vi "oa_TV Differentiator (1Chan).vi"(5 "reset? (True)":bool=TRUE, 8 "error in (no error)":errorcluster, 10 "deltaX":dbl=1.0 format="%.2f", 11 "Y[n]":dbl[](array[numeric]) format="%.2f") -> (0 "error out":errorcluster, 1 "Delay":dbl, 2 "X[n]":dbl[](array[numeric]) format="%.2f", 3 "dY[n]/dX[n]":dbl[](array[numeric]) format="%.2f")   [LabVIEW 2017, in "SoundVib_Torsional.lvlib"]
uses:
  <vilib>/addons/Sound and Vibration/Order Analysis/Torsional Vibration/SoundVib_Torsional.lvlib
  <vilib>/Analysis/3filter.llb/FIR Filter with I.C. (DBL).vi
  <vilib>/Analysis/NI_AALBase.lvlib
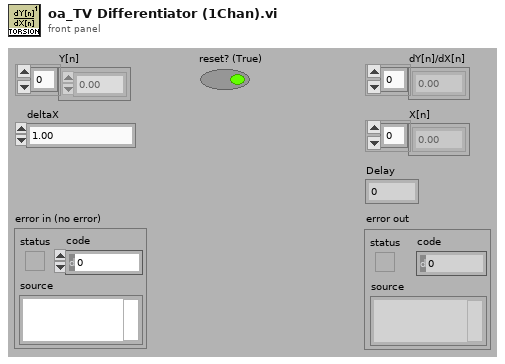
[diagram p1: front panel]
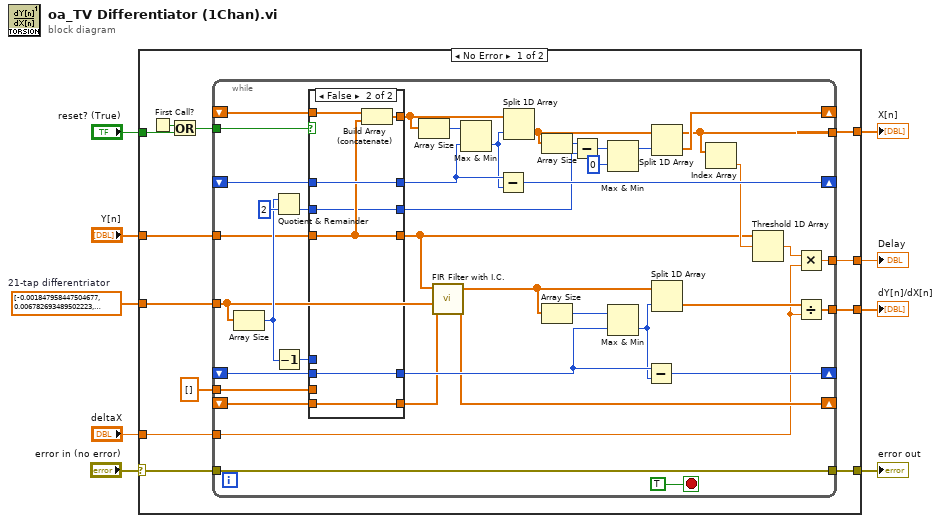
[diagram p0: block diagram]
diagram:
  w3 = dbl[] [-0.001847958447504677, 0.006782693489502223, -0.015759314785292692, 0.03157696398653407, -0.05723345514019107, 0.09716912388312568, -0.15901162473423236, 0.2593879138454093, -0.4476586474107506, 0.9725301910180191, 0.0, -0.9725301910180191, 0.4476586474107506, -0.2593879138454093, 0.15901162473423236, -0.09716912388312568, 0.05723345514019107, -0.03157696398653407, 0.015759314785292692, -0.006782693489502223, 0.001847958447504677]  # 21-tap differentriator
  n1 = case shown="No Error" "error in (no error)" {
    selector: "error in (no error)" -> [w20 w75]
    tunnel: [w17 w75] -> w9
    tunnel: [w21 _] -> w8
    tunnel: [w13 _] -> w7
    tunnel: "Y[n]" -> [w12 _]
    tunnel: w3 -> [w19 _]
    tunnel: "reset? (True)" -> [w16 _]
    tunnel: [w11 0.0] -> w2
    tunnel: "deltaX" -> [w10 _]
    frame No Error {
      n2 = First Call?() -> (First Call?: T/F=w15:bool)
      n3 = Or(x=w15, y=w16) -> (x .or. y?=w14:bool)
      n4 = while {
        tunnel: [w62] -> w21
        tunnel: w20 -> [w31]
        tunnel: w19 -> [w35]
        shift-right: [w32] -> _
        shift-left: _ -> [w60]
        shift-right: [w49] -> _
        shift-left: _ -> [w47]
        shift-right: [w55] -> _
        shift-left: _ -> [w54]
        tunnel: w14 -> [w30]
        tunnel: [w25] -> w13
        shift-right: [w40] -> _
        shift-left: _ -> [w45]
        tunnel: dbl[] [] ("t") -> [w37]
        tunnel: [w31] -> w17
        tunnel: w12 -> [w33]
        tunnel: [w23] -> w11
        tunnel: w10 -> [w22]
        stop <- TRUE stop-if-true
        n5 = Array Size(array=w35) -> (size(s)=w39:i32)
        n6 = Quotient & Remainder(x=w39, y=2) -> (floor(x/y)=w36:i32)  [unwired: 1 out]
        n7 = Decrement(x=w39) -> (x-1=w46:i32)
        n8 = case shown="False" w30 {
          tunnel: w60 -> [_ w71]
          tunnel: [w63 w69] -> w57
          tunnel: w54 -> [_ w69]
          tunnel: [w64 w73] -> w48
          tunnel: w47 -> [_ w72]
          tunnel: w46 -> [w66 _]
          tunnel: w45 -> [_ w70]
          tunnel: [w66 w70] -> w42
          tunnel: w37 -> [w65 _]
          tunnel: w36 -> [w63 w67]
          tunnel: [w65 w71] -> w34
          tunnel: w33 -> [w64 w68]
          tunnel: [w64 w68] -> w26
          tunnel: [w63 w67] -> w29
          frame True {
          }
          frame False {
            n9 = Build Array (concatenate)(w72, w68) -> (w73:dbl[])
          }
        }
        n10 = Array Size(array=w48) -> (size(s)=w58:i32)
        n11 = call-poly <vilib>:"FIR Filter with I.C..vi"("Initial X Conditions"=w34, "FIR Coefficients"=w35, "X"=w26) -> ("Final X Conditions"=w32:dbl[], "Filtered X"=w28:dbl[])  [unwired: 5 in, 1 out]
        n12 = Max & Min(x=w58, y=w57) -> (min(x,y)=w56:i32)  [unwired: 1 out]
        n13 = Subtract(x=w57, y=w56) -> (x-y=w55:i32)
        n14 = Split 1D Array(array=w48, index=w56) -> (second subarray=w53:dbl[])  [unwired: 1 out]
        n15 = Array Size(array=w53) -> (size(s)=w52:i32)
        n16 = Array Size(array=w28) -> (size(s)=w44:i32)
        n17 = Subtract(x=w52, y=w29) -> (x-y=w51:i32)
        n18 = Max & Min(x=w51, y=0) -> (max(x,y)=w38:i32)  [unwired: 1 out]
        n19 = Max & Min(x=w44, y=w42) -> (min(x,y)=w41:i32)  [unwired: 1 out]
        n20 = Subtract(x=w42, y=w41) -> (x-y=w40:i32)
        n21 = Split 1D Array(array=w53, index=w38) -> (first subarray=w25:dbl[], second subarray=w49:dbl[])
        n22 = Split 1D Array(array=w28, index=w41) -> (second subarray=w43:dbl[])  [unwired: 1 out]
        n23 = Index Array(array=w25) -> (element=w27:dbl)  [unwired: 1 in]
        n24 = Threshold 1D Array(2:w27, 3:w26) -> (0:w24:dbl)  [unwired: 1 in]
        n25 = Multiply(x=w24, y=w22) -> (x*y=w23:dbl)
        n26 = Divide(x=w43, y=w22) -> (x/y=w62:dbl[])
      }
    }
    frame Error {
    }
  }
  "dY[n]/dX[n]" <- w8
  "error out" <- w9
  "X[n]" <- w7
  "Delay" <- w2
